vi "WaitDIGIN.vi"(8 "error in (no error)":errorcluster, 9 "timeout (ms) default: 10s":i32=10000, 10 "Trigger default: board0 (t = 0)":T1, 11 "FPGA VI Reference In":refnum<k20>) -> (0 "error out":errorcluster, 1 "timeout?":bool, 2 "TriggerFired?":bool, 3 "FPGA VI Reference Out":refnum<k20>)   [LabVIEW 2014]
uses:
  TriggerChannel.ctl
  BLV/f_main_2014.vi
  <vilib>/rvi/interface/nirviReadWriteControl/nirviReadWriteControl.xnode
  NiFpgaLv.dll
  <vilib>/Utility/error.llb/Error Cluster From Error Code.vi
  <vilib>/rvi/errors/niLvFpgaAdjustHostInterfaceError.vi
  BLV/FPGA Bitfiles/W7XBolo_FPGATarget_fmain2014_oOwO-XGYwcQ.lvbitx
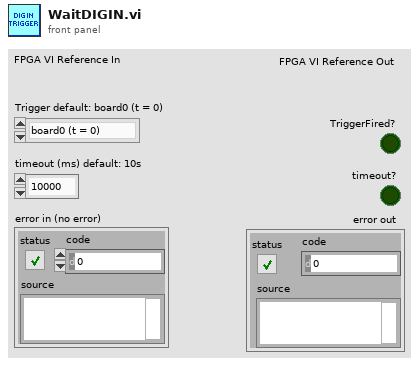
[diagram p1: front panel]
types:
  T1 = typedef "TriggerChannel.ctl" = enum16{"board0 (t = 0)", "board1 (t = -1min)", "board2 (t = -10sec)"}
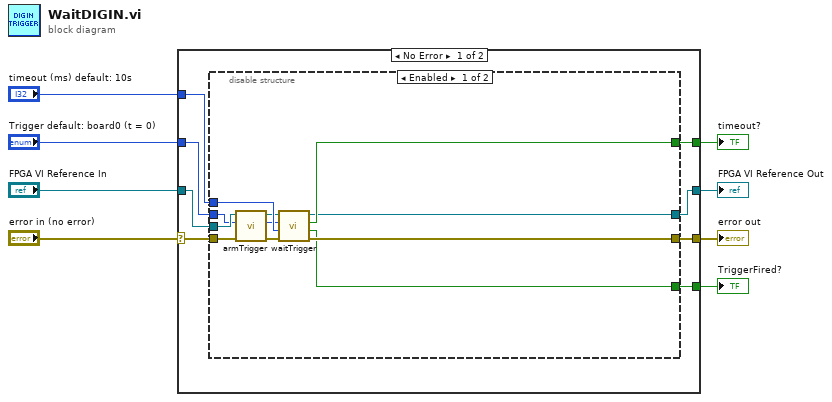
[diagram p0: block diagram]
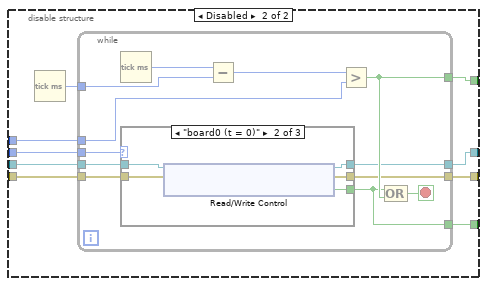
[diagram p2: hidden frame]
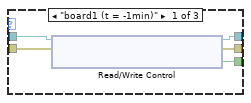
[diagram p3: hidden frame]
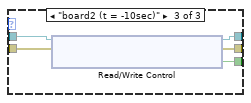
[diagram p4: hidden frame]
diagram:
  n1 = case shown="No Error" "error in (no error)" {
    selector: "error in (no error)" -> [w13 w65]
    tunnel: "timeout (ms) default: 10s" -> [w15 _]
    tunnel: [w12 w65] -> w7
    tunnel: "Trigger default: board0 (t = 0)" -> [w9 _]
    tunnel: [w16 _] -> w3
    tunnel: [w10 _] -> w4
    tunnel: "FPGA VI Reference In" -> [w14 w64]
    tunnel: [w11 w64] -> w1
    frame No Error {
      n2 = disable-structure shown="Enabled" {
        disable-tunnel: [w27 w33] -> w16
        disable-tunnel: w15 -> [w26 w34]
        disable-tunnel: w14 -> [w25 w31]
        disable-tunnel: w13 -> [w24 w29]
        disable-tunnel: [w23 w30] -> w12
        disable-tunnel: [w22 w28] -> w11
        disable-tunnel: [w21 w32] -> w10
        disable-tunnel: w9 -> [w18 w36]
        frame Enabled {
          n3 = call "armTrigger.vi"("error in (no error)"=w24, "Trigger default: board0 (t = 0)"=w18, "Refnum in"=w25) -> ("error out"=w20:errorcluster, "IRQ"=w17:i32, "Refnum out"=w19:refnum<k20>)  [unwired: 6 in]
          n4 = call "waitTrigger.vi"("error in (no error)"=w20, "timeout (ms) default: 10s"=w26, "IRQ"=w17, "Refnum in"=w19) -> ("error out"=w23:errorcluster, "Boolean"=w21:bool, "Timed Out"=w27:bool, "Refnum out"=w22:refnum<k20>)  [unwired: 4 in]
        }
        frame Disabled {
          n5 = Tick Count (ms)() -> (millisecond timer value=w35:u32)
          n6 = while {
            tunnel: w36 -> [w48]
            tunnel: w35 -> [w46]
            tunnel: w34 -> [w44]
            tunnel: [w42] -> w33
            tunnel: [w37] -> w32
            tunnel: w31 -> [w41]
            tunnel: [w40] -> w30
            tunnel: w29 -> [w39]
            tunnel: [w38] -> w28
            stop <- w43 stop-if-true
            n7 = Tick Count (ms)() -> (millisecond timer value=w47:u32)
            n8 = case shown="\"board0 (t = 0)\"" w48 {
              tunnel: w41 -> [w53 w58 w63]
              tunnel: [w52 w57 w62] -> w40
              tunnel: w39 -> [w51 w56 w61]
              tunnel: [w49 w54 w60] -> w38
              tunnel: [w50 w55 w59] -> w37
              frame "board1 (t = -1min)" {
                n9 = xnode "Read/Write Control"("FPGA VI Reference In"=w53, "error in"=w51) -> ("FPGA VI Reference Out"=w49:refnum<k20>, "error out"=w52:errorcluster, "C1DIGIN"=w50:bool)
              }
              frame "board0 (t = 0)" {
                n10 = xnode "Read/Write Control"("FPGA VI Reference In"=w58, "error in"=w56) -> ("FPGA VI Reference Out"=w54:refnum<k20>, "error out"=w57:errorcluster, "C0DIGIN"=w55:bool)
              }
              frame "board2 (t = -10sec)" {
                n11 = xnode "Read/Write Control"("FPGA VI Reference In"=w63, "error in"=w61) -> ("FPGA VI Reference Out"=w60:refnum<k20>, "error out"=w62:errorcluster, "C2DIGIN"=w59:bool)
              }
            }
            n12 = Subtract(x=w47, y=w46) -> (x-y=w45:u32)
            n13 = Greater?(x=w45, y=w44) -> (0:w42:bool)
            n14 = Compound Arithmetic op=OR(w37, w42) -> (w43:bool)
          }
        }
      }
    }
    frame Error {
    }
  }
  "error out" <- w7
  "TriggerFired?" <- w4
  "timeout?" <- w3
  "FPGA VI Reference Out" <- w1
